vi "Autodiscover Groups.vi"(8 "error in (no error)":errorcluster, 10 "Groups":T1[](array[typedef]), 11 "RemoteDataService in":refnum<class "RemoteDataService.lvclass">) -> (0 "error out":errorcluster, 3 "RemoteDataService out":refnum<class "RemoteDataService.lvclass">)   [LabVIEW 2020, in "Vecto.lvlib" / "RemoteDataService.lvclass"]
uses:
  RemoteDataService.lvclass
  proto/Discovery/Data.ctl
  proto/Service/Data.ctl
  proto/ServiceType/Enumeration.ctl
  RemoteDataService.lvclass/RemoteDataService.ctl
  proto/ServiceType/ServiceType.lvlib
  proto/Service/Service.lvlib
  proto/Discovery/Discovery.lvlib
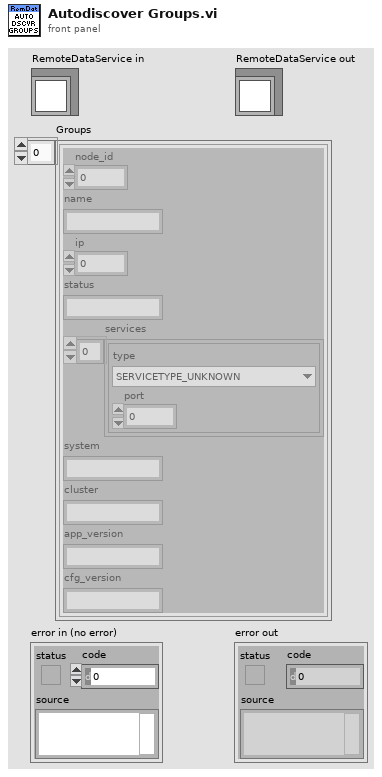
[diagram p1: front panel]
types:
  T1 = typedef "Discovery.lvlib/Data.ctl" = cluster{"node_id":u32, "name":string, "ip":u32, "status":string, "services":T2[], "system":string, "cluster":string, "app_version":string, "cfg_version":string}
  T2 = typedef "Service.lvlib/Data.ctl" = cluster{"type":T3, "port":i32}
  T3 = typedef "ServiceType.lvlib/Enumeration.ctl" = enum16{"SERVICETYPE_UNKNOWN", "SERVICETYPE_TCPSERVER", "SERVICETYPE_HTTPSERVER"}
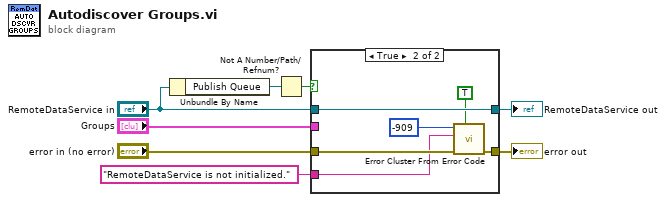
[diagram p0: block diagram]
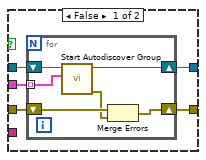
[diagram p2: hidden frame]
diagram:
  n1 = Unbundle By Name("RemoteDataService in") -> ("Publish Queue"=w3:refnum<queue>)
  n2 = Not A Number/Path/Refnum?(number/path/refnum=w3) -> (NaN/Path/Refnum?=w2:bool)
  n3 = case shown="True" w2 {
    tunnel: "Groups" -> [w13 _]
    tunnel: [w12 w25] -> w7
    tunnel: "error in (no error)" -> [w11 w23]
    tunnel: [w10 w24] -> w5
    tunnel: "RemoteDataService in" -> [w9 w25]
    tunnel: "RemoteDataService is not initialized." -> [_ w20]
    frame False {
      n4 = for {
        shift-right: [w17] -> w12
        shift-left: w9 -> [w19]
        tunnel: w13 -> [w18] mode=indexing
        shift-right: [w14] -> w10
        shift-left: w11 -> [w16]
        n5 = call "Start Autodiscover Group.vi"("Discovery"=w18, "RemoteDataService in"=w19) -> ("error out"=w15:errorcluster, "RemoteDataService out"=w17:refnum<class "RemoteDataService.lvclass">)  [unwired: 8 in]
        n6 = Merge Errors(w16, w15) -> (w14:errorcluster)
      }
    }
    frame True {
      n7 = call <vilib>:"Error Cluster From Error Code.vi"("show call chain? (False)"=TRUE, "error in (no error)"=w23, "error message (\"\")"=w20, "error code (0)"=-909) -> ("error out"=w24:errorcluster)  [unwired: 5 in]
    }
  }
  "error out" <- w5
  "RemoteDataService out" <- w7
